vi "make_installer_exe_custom.vi"(4 "config_value":T2, 6 "config_include":T1, 8 "error in (no error)":errorcluster, 10 "installer_directory":path, 11 "setup_filename in":path) -> (0 "error out":errorcluster, 3 "setup_filename out":path)   [LabVIEW 2015, in "lv-bin-7zip.lvlib" / "v1.lvlib"]
uses:
  v1.lvlib
  lv-bin-7zip.lvlib
  _controls/config_value.ctl
  _controls/config_include.ctl
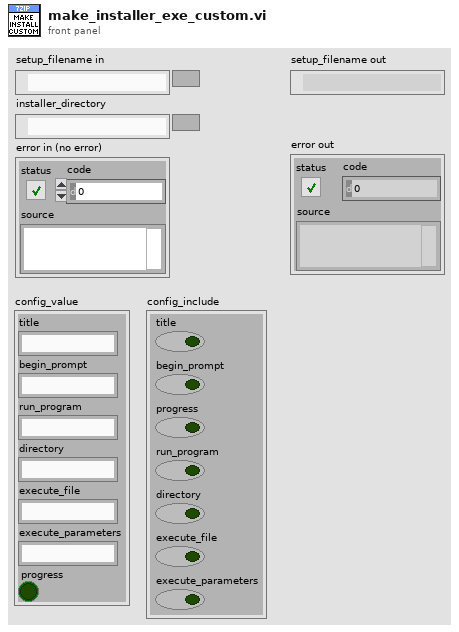
[diagram p1: front panel]
types:
  T1 = typedef "lv-bin-7zip.lvlib/v1.lvlib/config_include.ctl" = cluster{"title":bool, "begin_prompt":bool, "progress":bool, "run_program":bool, "directory":bool, "execute_file":bool, "execute_parameters":bool}
  T2 = typedef "lv-bin-7zip.lvlib/v1.lvlib/config_value.ctl" = cluster{"title":string, "begin_prompt":string, "run_program":string, "directory":string, "execute_file":string, "execute_parameters":string, "progress":bool}
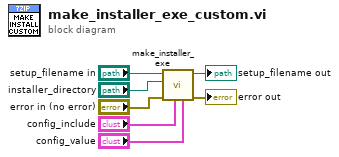
[diagram p0: block diagram]
diagram:
  n1 = call "make_installer_exe.vi"("config_value"="config_value", "config_include"="config_include", "error in (no error)"="error in (no error)", "installer_directory"="installer_directory", "setup_filename in"="setup_filename in") -> ("error out"=→"error out":errorcluster, "setup_filename out"=→"setup_filename out":path)  [unwired: 5 in]
